vi "ThermalStorage.vi"(5 "Day of Year":u32, 6 "Unique Object Identifier":string, 7 "Day Time":u32, 8 "Error In":errorcluster, 10 "Energy flow IN":T2, 11 "DataFlowIN":T1) -> (0 "Error Out":errorcluster, 2 "Energy flow OUT":T2, 3 "DataFlowOUT":T1)   [LabVIEW 2017]
uses:
  classes/DataCollector.lvclass
  classes/DataHandler.lvclass
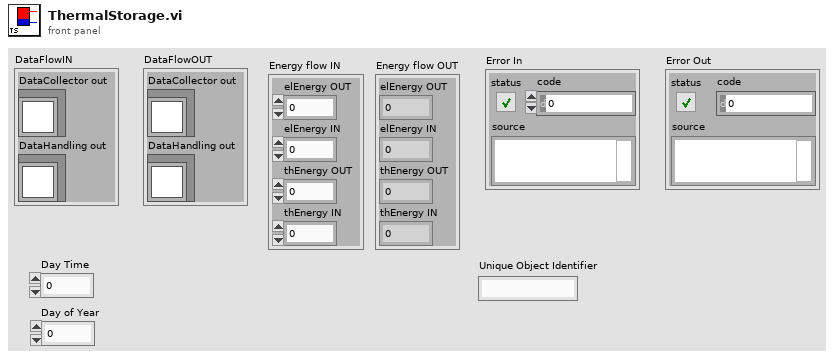
[diagram p1: front panel]
types:
  T1 = cluster{"DataCollector out":refnum<class "DataCollector.lvclass">, "DataHandling out":refnum<class "DataHandler.lvclass">}
  T2 = cluster{"elEnergy OUT":dbl, "elEnergy IN":dbl, "thEnergy OUT":dbl, "thEnergy IN":dbl}
  T3 = cluster{"Day Time":u32, "Day of Year":u32, "Energy flow IN":cluster{"elEnergy OUT":dbl, "elEnergy IN":dbl, "thEnergy OUT":dbl, "thEnergy IN":dbl}}
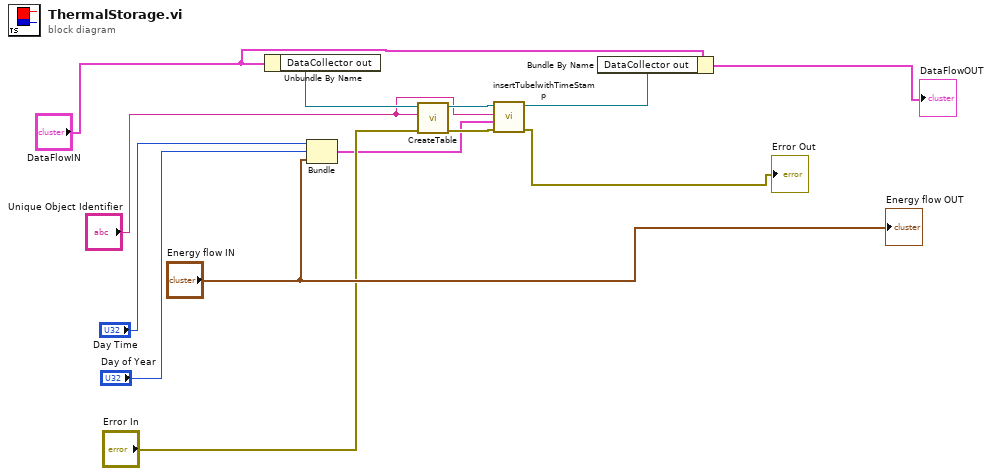
[diagram p0: block diagram]
diagram:
  n1 = Unbundle By Name("DataFlowIN") -> ("DataCollector out"=w13:refnum<class "DataCollector.lvclass">)
  n2 = Bundle("Day Time"="Day Time", "Day of Year"="Day of Year", "Energy flow IN"="Energy flow IN") -> (w2:T3)  [unwired: 1 in]
  n3 = call "CreateTable.vi"("error in (no error)"="Error In", "Name of Table"="Unique Object Identifier", "DataCollector in"=w13) -> ("error out"=w12:errorcluster, "DataCollector out"=w11:refnum<class "DataCollector.lvclass">)  [unwired: 7 in]
  n4 = call-dynamic "insertTubelwithTimeStamp.vi"("error in (no error)"=w12, "Data Cluster"=w2, "Name of Table"="Unique Object Identifier", "DataCollector in"=w11) -> ("error out"=→"Error Out":errorcluster, "DataCollector out"=w10:refnum<class "DataCollector.lvclass">)  [unwired: 6 in]
  n5 = Bundle By Name(cluster="DataFlowIN", "DataCollector out"=w10) -> (→"DataFlowOUT":T1)
  "Energy flow OUT" <- "Energy flow IN"
